vi "Learn_PFPC.vi"(8 "error in (no error)":errorcluster, 10 "CF Input":dbl, 11 "CNN in":refnum<class "CNN.lvclass">) -> (0 "error out":errorcluster, 3 "CNN out":refnum<class "CNN.lvclass">)   [LabVIEW 2016, in "CNN.lvclass"]
uses:
  CNN.lvclass
  CNN.lvclass/CNN.ctl
panel:
  out "WPFPC":dbl[](graph)
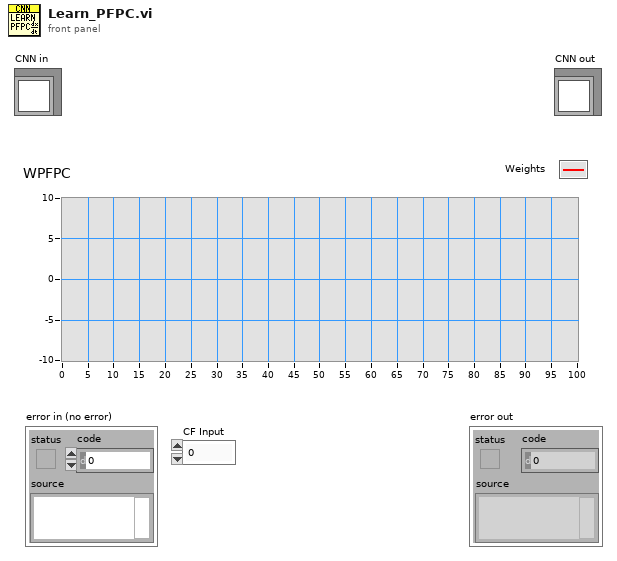
[diagram p1: front panel]
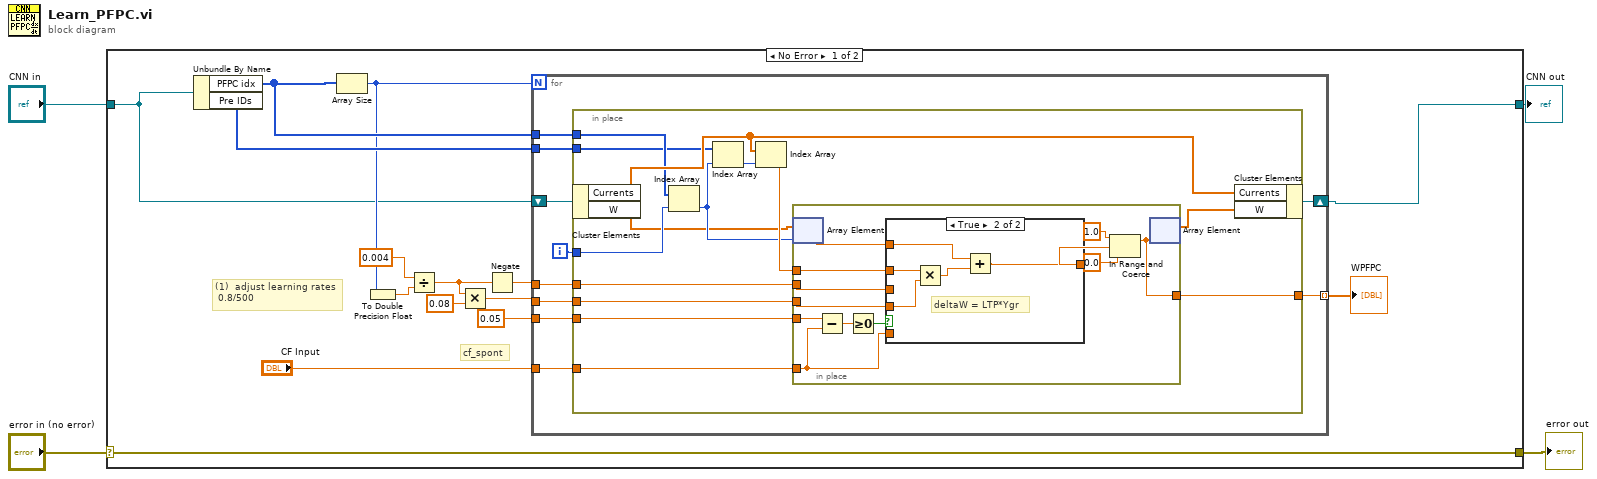
[diagram p0: block diagram]
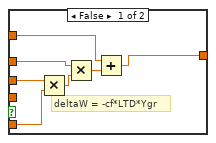
[diagram p2: hidden frame]
diagram:
  n1 = case shown="No Error" "error in (no error)" {
    selector: "error in (no error)" -> [w19 w68]
    tunnel: [w19 w68] -> w3
    tunnel: [w6 w69] -> w1
    tunnel: "CNN in" -> [w5 w69]
    frame No Error {
      # "cf_spont"
      # "(1)  adjust learning rates\n 0.8/500"
      n2 = Unbundle By Name(w5) -> ("PFPC idx"=w17:i32[], "Pre IDs"=w16:i32[])
      n3 = Array Size(array=w17) -> (size(s)=w11:i32)
      n4 = To Double Precision Float(number=w11) -> (double precision float=w8:dbl)
      n5 = Divide(x=0.004, y=w8) -> (x/y=w14:dbl)
      n6 = Multiply(x=w14, y=0.08) -> (x*y=w12:dbl)
      n7 = Negate(x=w14) -> (-x=w13:dbl)
      n8 = for {
        N: w11 -> [_]
        shift-right: [w29] -> w6
        shift-left: w5 -> [w25]
        tunnel: "CF Input" -> [w28]
        tunnel: w12 -> [w27]
        tunnel: 0.05 ("x") -> [w26]
        tunnel: w13 -> [w23]
        tunnel: w17 -> [w22]
        tunnel: w16 -> [w21]
        tunnel: [w20] -> w7 mode=indexing
        i -> [w24]
        n9 = in-place {
          in-place-border: w28 -> [w43]
          in-place-border: w27 -> [w39]
          in-place-border: w26 -> [w42]
          in-place-border: w24 -> [w35]
          in-place-border: w23 -> [w38]
          in-place-border: w22 -> [w34]
          in-place-border: w21 -> [w33]
          in-place-border: [w30] -> w20
          n10 = in-place-cluster #1(w25) -> ("Currents"=w40:dbl[], "W"=w32:dbl[])
          n11 = Index Array(array=w34, index=w35) -> (element=w37:i32)
          n12 = Index Array(array=w33, index=w37) -> (element=w36:i32)
          n13 = Index Array(array=w40, index=w36) -> (element=w41:dbl)
          n14 = in-place {
            in-place-border: w43 -> [w49]
            in-place-border: w41 -> [w53]
            in-place-border: w42 -> [w55]
            in-place-border: w39 -> [w52]
            in-place-border: w38 -> [w51]
            in-place-border: [w44] -> w30
            n15 = in-place-array #2(w32, w37) -> (w48:dbl)
            n16 = Subtract(x=w55, y=w49) -> (x-y=w50:dbl)
            n17 = Greater Or Equal To 0?(x=w50) -> (x >= 0?=w54:bool)
            n18 = case shown="True" w54 {
              tunnel: w48 -> [w62 w67]
              tunnel: [w56 w63] -> w45
              tunnel: w53 -> [w61 w66]
              tunnel: w52 -> [_ w65]
              tunnel: w51 -> [w58 _]
              tunnel: w49 -> [w60 _]
              frame False {
                # "deltaW = -cf*LTD*Ygr"
                n19 = Multiply(x=w58, y=w60) -> (x*y=w59:dbl)
                n20 = Multiply(x=w61, y=w59) -> (x*y=w57:dbl)
                n21 = Add(x=w62, y=w57) -> (x+y=w56:dbl)
              }
              frame True {
                # "deltaW = LTP*Ygr"
                n22 = Multiply(x=w66, y=w65) -> (x*y=w64:dbl)
                n23 = Add(x=w67, y=w64) -> (x+y=w63:dbl)
              }
            }
            n24 = In Range and Coerce(upper limit=1.0, x=w45, lower limit=0.0) -> (coerced(x)=w44:dbl)  [unwired: 1 out]
            n25 = in-place-array #2(w44) -> (w31:dbl[])  [unwired: 1 out]
          }
          n26 = in-place-cluster #1("Currents"=w40, "W"=w31) -> (w29:refnum<class "CNN.lvclass">)
        }
      }
      "WPFPC" <- w7
    }
    frame Error {
    }
  }
  "error out" <- w3
  "CNN out" <- w1
